vi "Attach To Process.vi"(8 "error in (no error)":errorcluster, 10 "Process In":refnum<class "Process.lvclass">, 11 "Broadcast Message Receiver In":refnum<class "Broadcast Message Receiver.lvclass">) -> (0 "error out":errorcluster, 3 "Broadcast Message Receiver Out":refnum<class "Broadcast Message Receiver.lvclass">)   [LabVIEW 2020, in "Broadcast Message Receiver.lvclass"]
uses:
  Broadcast Message Receiver.lvclass
  C:/Git/astemes-triarc-debugger/source/Process/Debug Process.lvclass
  Process/Debug Process.lvclass/Debug Process.ctl
  Broadcast Message Receiver.lvclass/Broadcast Message Receiver.ctl
  <vilib>/Utility/error.llb/Clear Errors.vi
  <vilib>/Utility/error.llb/Error Cluster From Error Code.vi
  C:/Git/astemes-triarc-debugger/source/Broadcast Message Receiver/Broadcast Message Receiver.lvclass
  Process/Debug Process.lvclass
  <vilib>/Astemes/Triarc Framework/Process/Process.lvclass
  C:/Program Files (x86)/National Instruments/LabVIEW 2020/vi.lib/Astemes/Triarc Framework/Base/Base.lvclass
  C:/Program Files (x86)/National Instruments/LabVIEW 2020/vi.lib/Astemes/Triarc Framework/Process/Process.lvclass
  C:/Program Files (x86)/National Instruments/LabVIEW 2020/vi.lib/Astemes/Triarc Framework/Error Handler Interface/Error Handler Interface.lvclass
  C:/Program Files (x86)/National Instruments/LabVIEW 2020/vi.lib/Astemes/Triarc Framework/Logging/Logging.lvclass
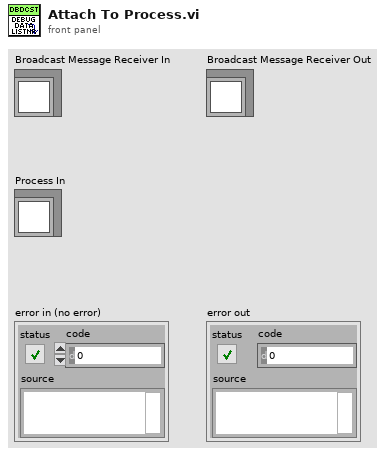
[diagram p1: front panel]
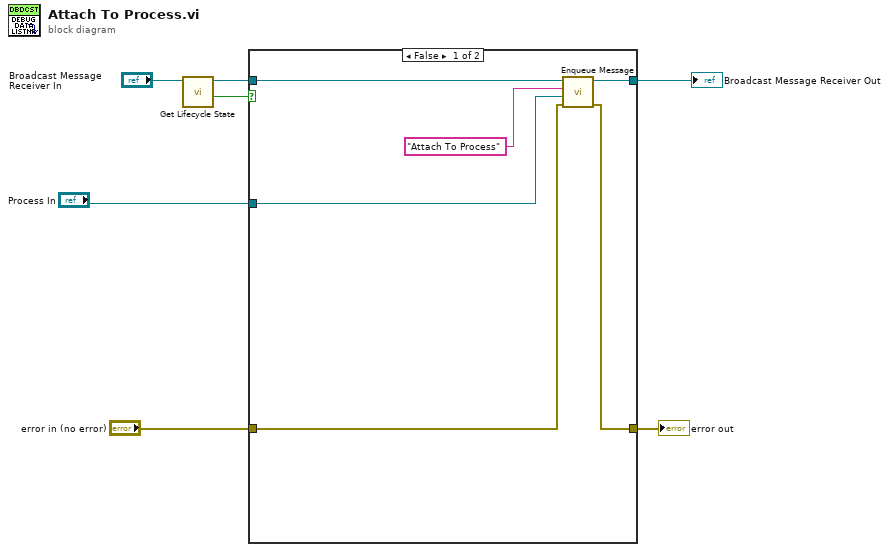
[diagram p0: block diagram]
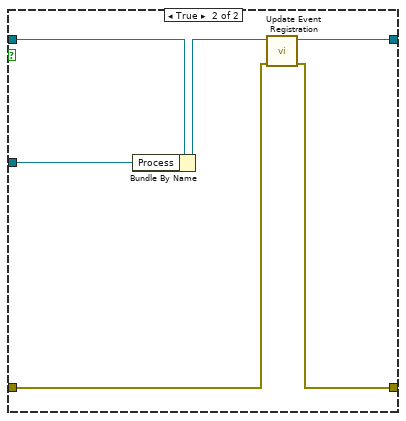
[diagram p2: hidden frame]
diagram:
  n1 = call "Get Lifecycle State.vi"("Process In"="Broadcast Message Receiver In") -> ("In Process Loop?"=w3:bool, "Process Out"=w6:refnum<class "Broadcast Message Receiver.lvclass">)  [unwired: 7 in, 2 out]
  n2 = case shown="False" w3 {
    tunnel: w6 -> [w13 w19]
    tunnel: [w12 w18] -> w5
    tunnel: "error in (no error)" -> [w8 w16]
    tunnel: [w9 w17] -> w4
    tunnel: "Process In" -> [w11 w14]
    frame False {
      n3 = call "Enqueue Message.vi"("error in (no error)"=w8, "Message Data"=w11, "Message"="Attach To Process" ("API Message"), "Process In"=w13) -> ("error out"=w9:errorcluster, "Process Out"=w12:refnum<class "Broadcast Message Receiver.lvclass">)  [unwired: 6 in]
    }
    frame True {
      n4 = Bundle By Name(cluster=w19, "Process"=w14) -> (w15:refnum<class "Broadcast Message Receiver.lvclass">)
      n5 = call "Update Event Registration.vi"("error in (no error)"=w16, "Broadcast Message Receiver in"=w15) -> ("error out"=w17:errorcluster, "Broadcast Message Receiver out"=w18:refnum<class "Broadcast Message Receiver.lvclass">)  [unwired: 8 in]
    }
  }
  "error out" <- w4
  "Broadcast Message Receiver Out" <- w5
